vi "(A) Test-Sequence-Control (SubVI).vi"(0 "TEST MODE":bool, 1 "START":bool, 2 "STOP":bool, 3 "Hold-Step?":bool, 4 "Command Next Step":bool, 5 "Step Control":T2={"Step Description"="Description", "Step Time Target"=10.0, "Step Time Unit"=0, "Step End Action"=0} {"Step End Action" items=["Go to Next Step", "Loop to 1st Step", "Loop to Step N", "Stop Test Mode", "Stop Program"]; "Step Time Target" min=0.0 format="%#.1f"; "Step Time Unit" items=["sec", "min", "hr"]}, 7 "Step # Limit":i32=50, 9 "Loop # Limit":i32=10, 11 "Step N":i32=3, 13 "Initialize":bool) -> (14 "Output Values":T1={"Manual-Mode-Active?"=FALSE, "Test-Mode-Active?"=FALSE, "STEP-COMPLETE"=FALSE, "Test Description"="Manual Mode - Press Start to Begin\r\r", "Step-Time"="", "Step Text"="", "Loop Text"="", "Step Number"=-1, "Loop Number"=0}, 15 "Display":string="Manual Mode - Press Start to Begin", 16 "Step Number":i32=-1, 17 "Loop Number":i32, 18 "TEST MODE ACTIVE?":bool, 19 "STOP-PROGRAM":bool)   [LabVIEW 2010]
panel:
  # "Blake Otting - Ecolab\nCreated 5/28/07\nUpdated 2/4/11 (Rev 10.3)"
  # "Step Time Target"
  # "Units"
  # "Step End Action"
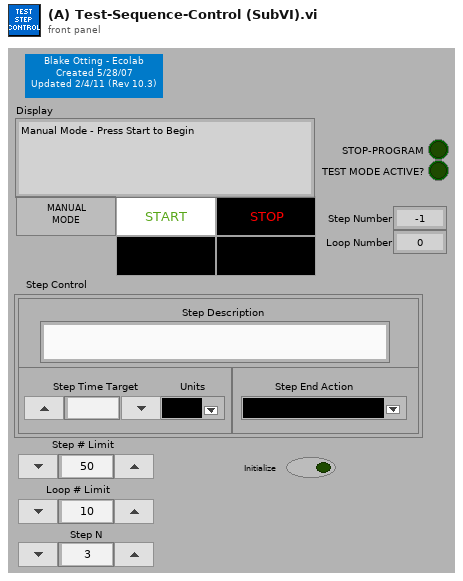
[diagram p1: front panel]
types:
  T1 = cluster{"Manual-Mode-Active?":bool, "Test-Mode-Active?":bool, "STEP-COMPLETE":bool, "Test Description":string, "Step-Time":string, "Step Text":string, "Loop Text":string, "Step Number":i32, "Loop Number":i32}
  T2 = cluster{"Step Description":string, "Step Time Target":dbl, "Step Time Unit":u16, "Step End Action":u16}
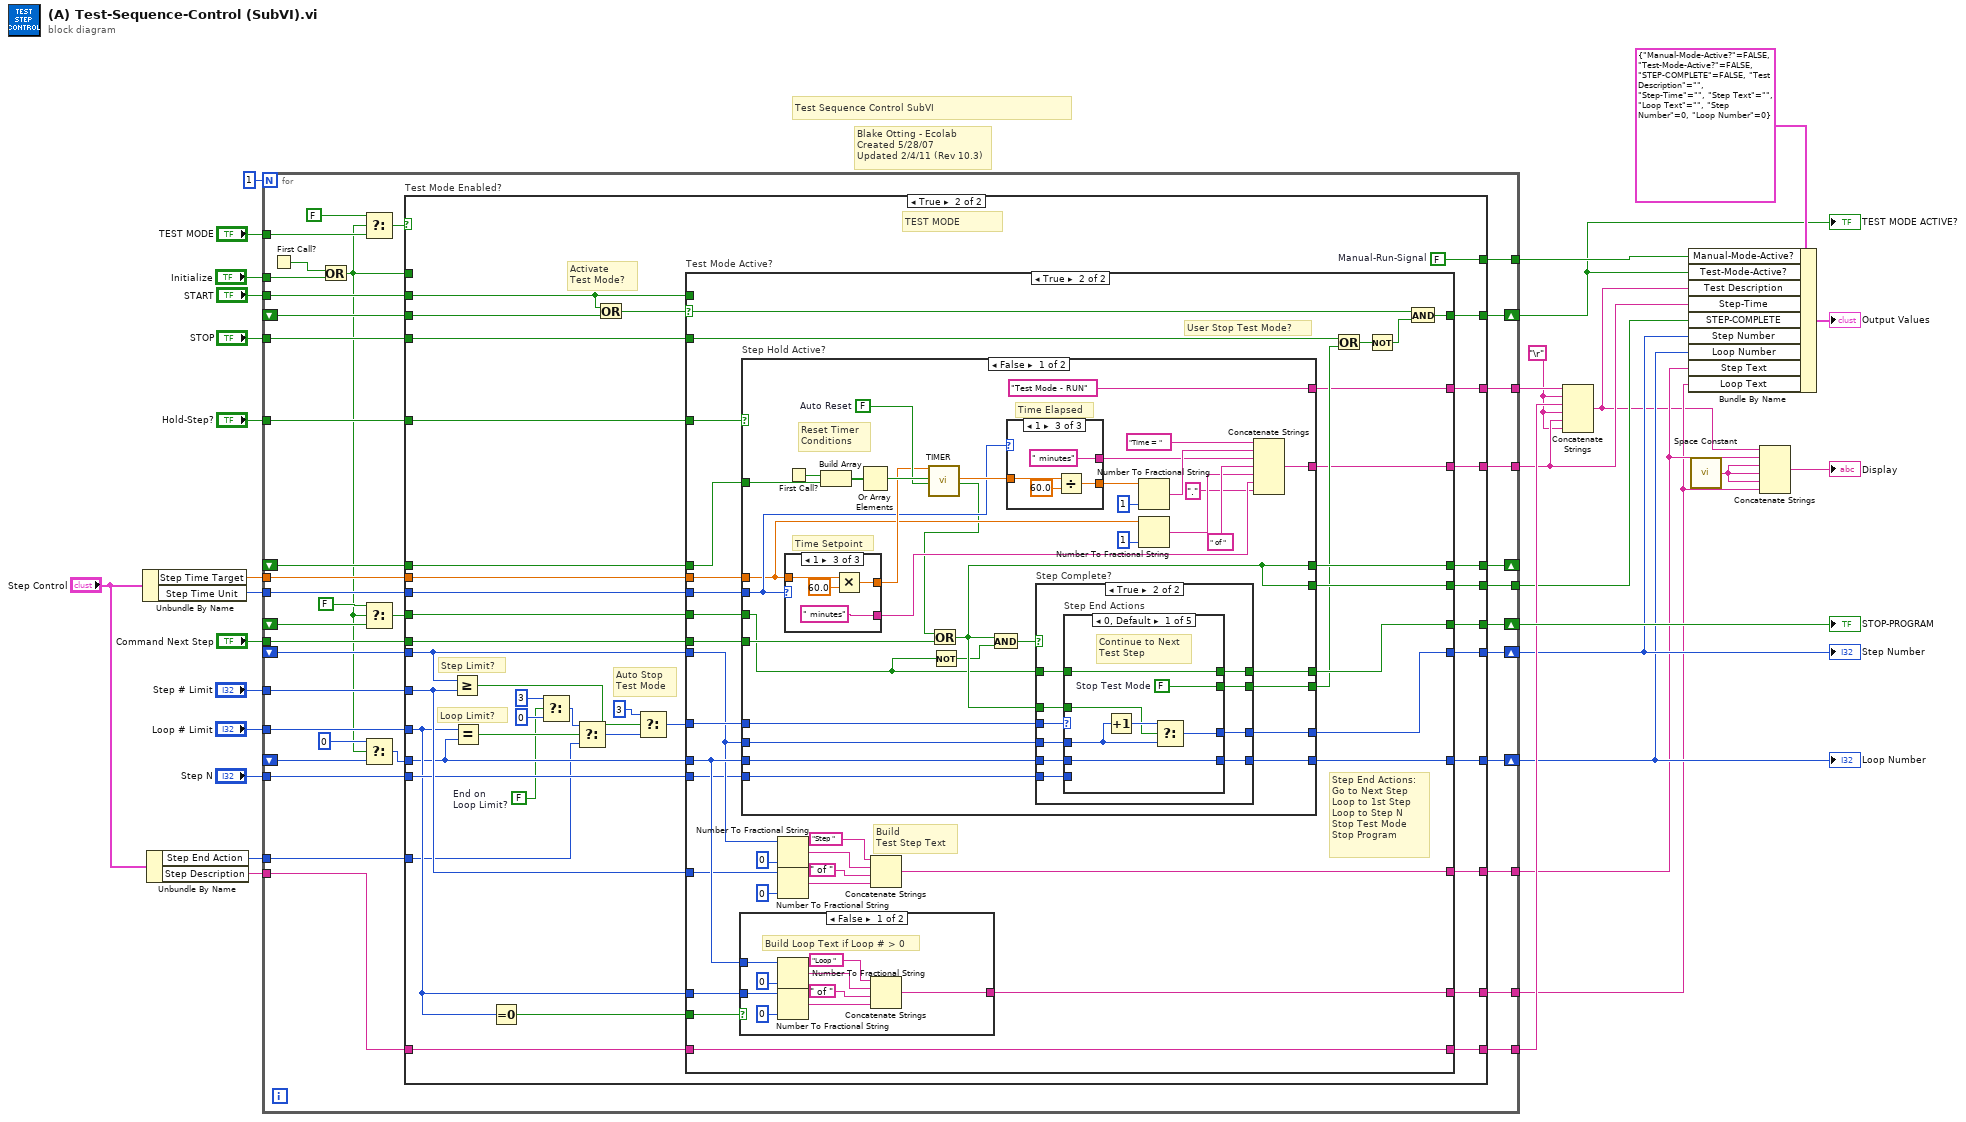
[diagram p0: block diagram]
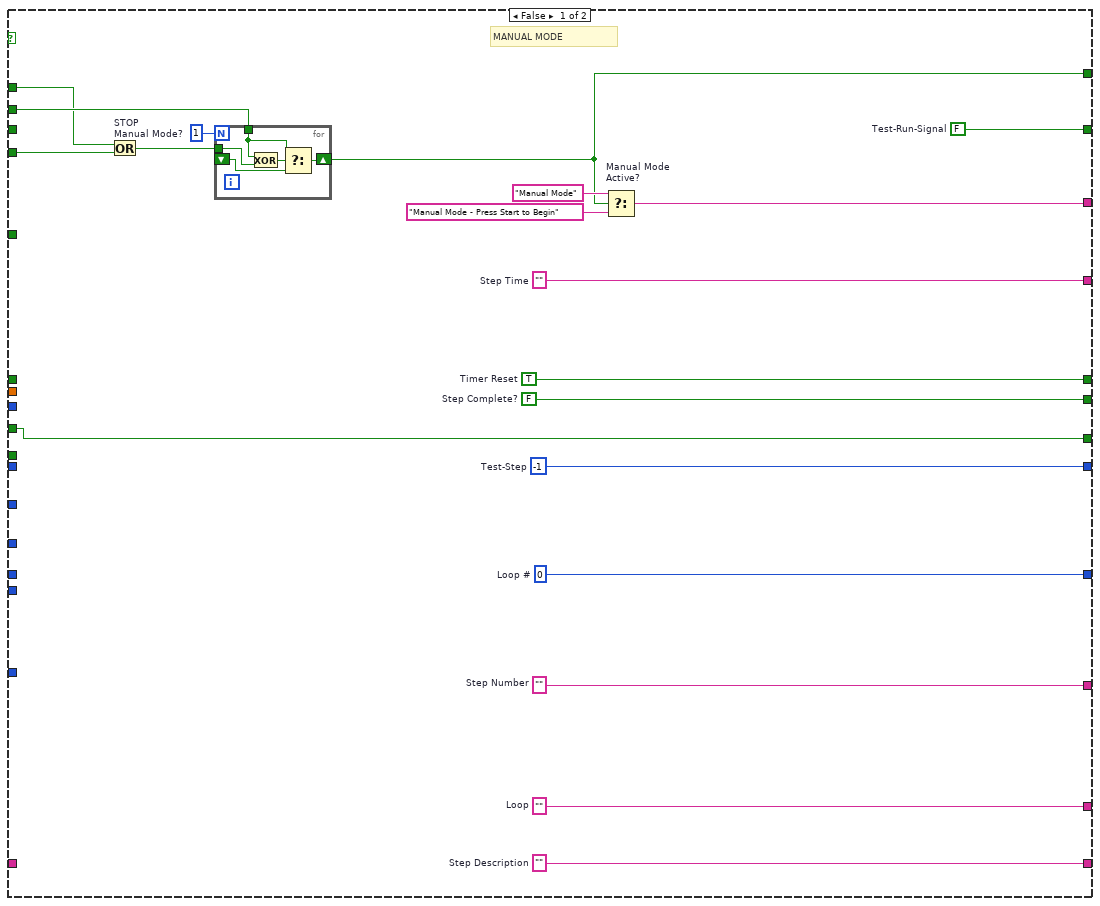
[diagram p2: hidden frame]
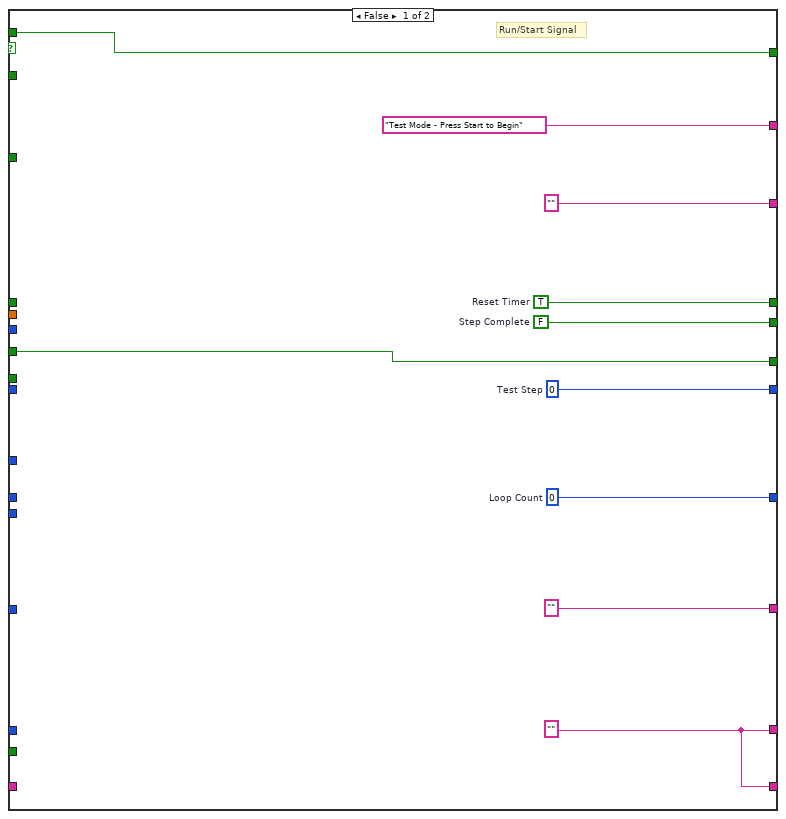
[diagram p3: hidden frame]
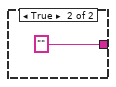
[diagram p4: hidden frame]
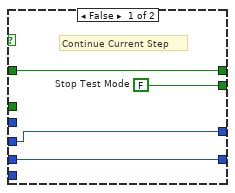
[diagram p5: hidden frame]
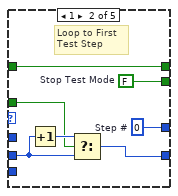
[diagram p6: hidden frame]
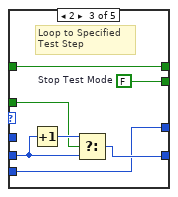
[diagram p7: hidden frame]
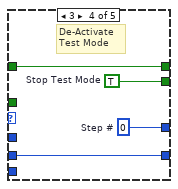
[diagram p8: hidden frame]
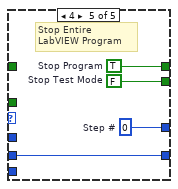
[diagram p9: hidden frame]
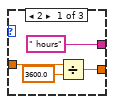
[diagram p10: hidden frame]
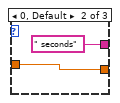
[diagram p11: hidden frame]
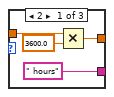
[diagram p12: hidden frame]
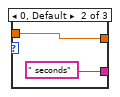
[diagram p13: hidden frame]
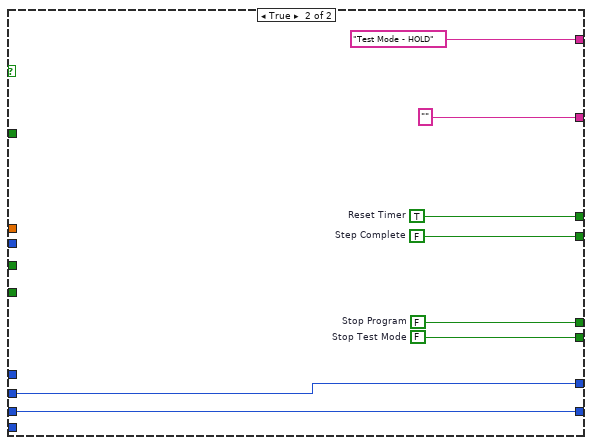
[diagram p14: hidden frame]
diagram:
  w4 = "\r"
  # "Test Sequence Control SubVI"
  # "Blake Otting - Ecolab\nCreated 5/28/07\nUpdated 2/4/11 (Rev 10.3)"
  n1 = Unbundle By Name("Step Control") -> ("Step Time Target"=w24:dbl, "Step Time Unit"=w25:u16)
  n2 = Unbundle By Name("Step Control") -> ("Step End Action"=w27:u16, "Step Description"=w26:string)
  n3 = for {
    N: 1 -> [_]
    tunnel: "Command Next Step" -> [w70]
    tunnel: [w69] -> w17
    tunnel: "TEST MODE" -> [w44]
    tunnel: "START" -> [w68]
    tunnel: "STOP" -> [w67]
    tunnel: [w65] -> w12
    tunnel: "Hold-Step?" -> [w64]
    tunnel: "Step # Limit" -> [w63]
    tunnel: "Loop # Limit" -> [w62]
    tunnel: [w61] -> w9
    tunnel: [w60] -> w3
    tunnel: [w59] -> w13
    tunnel: [w53] -> w23
    tunnel: w24 -> [w52]
    tunnel: w25 -> [w51]
    tunnel: w27 -> [w50]
    tunnel: w26 -> [w49]
    shift-right: [w55] -> w11
    shift-left: _ -> [w48]
    shift-right: [w54] -> w10
    shift-left: _ -> [w42]
    shift-right: [w56] -> _
    shift-left: _ -> [w47]
    shift-right: [w58] -> w14
    shift-left: _ -> [w46]
    tunnel: [w57] -> w15
    tunnel: "Step N" -> [w39]
    tunnel: "Initialize" -> [w35]
    shift-right: [w66] -> w21
    shift-left: _ -> [w37]
    n4 = First Call?() -> (First Call?: T/F=w34:bool)
    n5 = Or(x=w34, y=w35) -> (x .or. y?=w33:bool)
    n6 = Select(t=FALSE, s=w33, f=w44) -> (s? t:f=w43:bool)
    n7 = Select(t=FALSE, s=w33, f=w37) -> (s? t:f=w36:bool)
    n8 = Select(t=0, s=w33, f=w42) -> (s? t:f=w40:i32)
    n9 = case "Test Mode Enabled?" shown="True" w43 {
      tunnel: w68 -> [w78 w129]
      tunnel: w67 -> [w77 w132]
      tunnel: [w72 w133] -> w53
      tunnel: w46 -> [_ w131]
      tunnel: [w89 w130] -> w58
      tunnel: [w71 w127] -> w66
      tunnel: [w88 w126] -> w65
      tunnel: w64 -> [_ w125]
      tunnel: [w87 w124] -> w55
      tunnel: [w84 w123] -> w56
      tunnel: [w86 w122] -> w54
      tunnel: w63 -> [_ w119]
      tunnel: w62 -> [_ w105]
      tunnel: [w83 w118] -> w61
      tunnel: [w82 w117] -> w60
      tunnel: [w85 w116] -> w59
      tunnel: [w73 w115] -> w57
      tunnel: w47 -> [_ w114]
      tunnel: w48 -> [_ w113]
      tunnel: w40 -> [_ w104]
      tunnel: w52 -> [_ w112]
      tunnel: w51 -> [_ w111]
      tunnel: w50 -> [_ w102]
      tunnel: w49 -> [_ w110]
      tunnel: [w81 w109] -> w69
      tunnel: w70 -> [_ w108]
      tunnel: w33 -> [w76 _]
      tunnel: w39 -> [_ w107]
      tunnel: w36 -> [w71 w100]
      frame False {
        w81 = ""  # Step Description
        w82 = ""  # Loop
        w83 = ""  # Step Number
        w84 = TRUE  # Timer Reset
        w85 = ""  # Step Time
        w86 = 0  # Loop #
        w87 = -1  # Test-Step
        w88 = FALSE  # Step Complete?
        w89 = FALSE  # Test-Run-Signal
        # "MANUAL MODE"
        n10 = Or "STOP\nManual Mode?"(x=w76, y=w77) -> (x .or. y?=w80:bool)
        n11 = for {
          N: 1 -> [_]
          tunnel: w78 -> [w93]
          shift-right: [w91] -> w73
          shift-left: _ -> [w92]
          tunnel: w80 -> [w90]
          n12 = Exclusive Or(1:w90, 2:w93) -> (0:w94:bool)
          n13 = Select(t=w93, s=w94, f=w92) -> (s? t:f=w91:bool)
        }
        n14 = Select "Manual Mode\nActive?"(t="Manual Mode", s=w73, f="Manual Mode - Press Start to Begin") -> (s? t:f=w72:string)
      }
      frame True {
        w95 = FALSE  # End on Loop Limit?
        w115 = FALSE  # Manual-Run-Signal
        # "Loop Limit?"
        # "TEST MODE"
        # "Activate\nTest Mode?"
        # "Auto Stop\nTest Mode"
        # "Step Limit?"
        n15 = Greater Or Equal?(x=w113, y=w119) -> (x >= y?=w106:bool)
        n16 = Equal?(x=w105, y=w104) -> (x = y?=w103:bool)
        n17 = Equal To 0?(x=w105) -> (x = 0?=w120:bool)
        n18 = Select(t=u16 3, s=w95, f=u16 0) -> (s? t:f=w96:u16)
        n19 = Select(t=w96, s=w103, f=w102) -> (s? t:f=w101:u16)
        n20 = Or(x=w129, y=w131) -> (x .or. y?=w128:bool)
        n21 = Select(t=u16 3 ("element"), s=w106, f=w101) -> (s? t:f=w121:u16)
        n22 = case "Test Mode Active?" shown="True" w128 {
          selector: w128 -> [_ w178]
          tunnel: w132 -> [_ w167]
          tunnel: ["Test Mode - Press Start to Begin" w164] -> w133
          tunnel: [w142 w176] -> w130
          tunnel: w129 -> [w142 _]
          tunnel: w113 -> [_ w155]
          tunnel: [w134 w169] -> w127
          tunnel: [w141 w168] -> w126
          tunnel: w125 -> [_ w175]
          tunnel: [w140 w174] -> w124
          tunnel: [w136 w173] -> w123
          tunnel: [w139 w172] -> w122
          tunnel: w104 -> [_ w162]
          tunnel: w114 -> [_ w171]
          tunnel: w121 -> [_ w170]
          tunnel: w120 -> [_ w163]
          tunnel: w105 -> [_ w161]
          tunnel: w119 -> [_ w154]
          tunnel: ["" w153] -> w118
          tunnel: [w135 w151] -> w117
          tunnel: w112 -> [_ w150]
          tunnel: w111 -> [_ w149]
          tunnel: ["" w148] -> w116
          tunnel: w110 -> [_ w147]
          tunnel: [w135 w147] -> w109
          tunnel: w108 -> [_ w146]
          tunnel: w107 -> [_ w145]
          tunnel: w100 -> [w134 w144]
          frame False {
            w136 = TRUE  # Reset Timer
            w135 = ""
            w139 = 0  # Loop Count
            w140 = 0  # Test Step
            w141 = FALSE  # Step Complete
            # "Run/Start Signal"
          }
          frame True {
            # "Step End Actions:\nGo to Next Step\nLoop to 1st Step\nLoop to Step N\nStop Test Mode\nStop Program"
            # "Build \nTest Step Text"
            # "User Stop Test Mode?"
            n23 = case shown="False" w163 {
              tunnel: w162 -> [w185 _]
              tunnel: w161 -> [w183 _]
              tunnel: [w179 ""] -> w151
              frame False {
                # "Build Loop Text if Loop # > 0"
                n24 = Number To Fractional String(number=w185, precision (6)=i16 0 ("width (-)")) -> (F-format string=w184:string)  [unwired: 2 out]
                n25 = Number To Fractional String(number=w183, precision (6)=i16 0 ("width (-)")) -> (F-format string=w182:string)  [unwired: 2 out]
                n26 = Concatenate Strings("Loop ", w184, " of ", w182) -> (w179:string)
              }
              frame True {
              }
            }
            n27 = case "Step Hold Active?" shown="False" w175 {
              tunnel: [w223 w289] -> w174
              tunnel: [w193 w294] -> w173
              tunnel: [w193 w293] -> w168
              tunnel: w155 -> [w218 w289]
              tunnel: [w217 w292] -> w172
              tunnel: w162 -> [w216 w292]
              tunnel: w171 -> [w215 _]
              tunnel: w170 -> [w214 _]
              tunnel: [w213 w288] -> w169
              tunnel: [w212 w291] -> w166
              tunnel: ["Test Mode - RUN" "Test Mode - HOLD"] -> w164
              tunnel: w150 -> [w196 _]
              tunnel: w149 -> [w198 _]
              tunnel: [w197 ""] -> w148
              tunnel: w146 -> [w195 _]
              tunnel: w145 -> [w194 _]
              tunnel: w144 -> [w191 _]
              frame False {
                w221 = FALSE  # Auto Reset
                # "Time Elapsed"
                # "Time Setpoint"
                # "Reset Timer\nConditions"
                n28 = First Call?() -> (First Call?: T/F=w220:bool)
                n29 = case "Time Target & Units" shown="1" w198 {
                  tunnel: [" hours" " seconds" " minutes"] -> w200
                  tunnel: [w278 w281 w284] -> w206
                  tunnel: w196 -> [w279 w281 w285]
                  frame 2 {
                    n30 = Multiply(x=w279, y=3600.0) -> (x*y=w278:dbl)
                  }
                  frame 0, Default {
                  }
                  frame 1 {
                    n31 = Multiply(x=w285, y=60.0) -> (x*y=w284:dbl)
                  }
                }
                n32 = Build Array(w220, w215) -> (w219:bool[])
                n33 = Or Array Elements(Boolean array=w219) -> (logical OR=w222:bool)
                n34 = call "TIMER"("Time Target (s)"=w206, "Reset"=w222, "Auto Reset"=w221) -> ("Elapsed Time (s)"=w210:dbl, "Time has Elapsed"=w189:bool)  [unwired: 2 in, 13 out]
                n35 = Or(x=w189, y=w195) -> (x .or. y?=w193:bool)
                n36 = Not(x=w191) -> (.not. x?=w190:bool)
                n37 = And(x=w193, y=w190) -> (x .and. y?=w192:bool)
                n38 = case "Time Target & Units" shown="1" w198 {
                  tunnel: w210 -> [w270 w272 w276]
                  tunnel: [w268 w272 w274] -> w205
                  tunnel: [" hours" " seconds" " minutes"] -> w203
                  frame 2 {
                    n39 = Divide(x=w270, y=3600.0) -> (x/y=w268:dbl)
                  }
                  frame 0, Default {
                  }
                  frame 1 {
                    n40 = Divide(x=w276, y=60.0) -> (x/y=w274:dbl)
                  }
                }
                n41 = case "Step Complete?" shown="True" w192 {
                  tunnel: [w226 w237] -> w223
                  tunnel: w218 -> [w226 w236]
                  tunnel: [w225 w235] -> w217
                  tunnel: w216 -> [w225 w234]
                  tunnel: w214 -> [_ w233]
                  tunnel: [w224 w232] -> w213
                  tunnel: [w227 w231] -> w212
                  tunnel: w193 -> [_ w230]
                  tunnel: w194 -> [_ w229]
                  tunnel: w191 -> [w224 w228]
                  frame False {
                    w227 = FALSE  # Stop Test Mode
                    # "Continue Current Step"
                  }
                  frame True {
                    n42 = case "Step End Actions" shown="0, Default" w233 {
                      tunnel: [w241 w251 w253 w262 w265] -> w237
                      tunnel: [w238 w245 w252 w259 w266] -> w232
                      tunnel: [w240 w250 w256 w260 w263] -> w235
                      tunnel: w236 -> [w243 _ _ _ _]
                      tunnel: w230 -> [w242 w248 w255 _ _]
                      tunnel: w234 -> [w240 w247 w254 w260 w263]
                      tunnel: [w239 w246 w258 w261 w264] -> w231
                      tunnel: w229 -> [_ _ w253 _ _]
                      tunnel: w228 -> [w238 w245 w252 w259 _]
                      frame 0, Default {
                        w239 = FALSE  # Stop Test Mode
                        # "Continue to Next\nTest Step"
                        n43 = Increment(x=w243) -> (x+1=w244:i32)
                        n44 = Select(t=w244, s=w242, f=w243) -> (s? t:f=w241:i32)
                      }
                      frame 1 {
                        w246 = FALSE  # Stop Test Mode
                        w251 = 0  # Step #
                        # "Loop to First\nTest Step"
                        n45 = Increment(x=w247) -> (x+1=w249:i32)
                        n46 = Select(t=w249, s=w248, f=w247) -> (s? t:f=w250:i32)
                      }
                      frame 2 {
                        w258 = FALSE  # Stop Test Mode
                        # "Loop to Specified\nTest Step"
                        n47 = Increment(x=w254) -> (x+1=w257:i32)
                        n48 = Select(t=w257, s=w255, f=w254) -> (s? t:f=w256:i32)
                      }
                      frame 3 {
                        w261 = TRUE  # Stop Test Mode
                        w262 = 0  # Step #
                        # "De-Activate \nTest Mode"
                      }
                      frame 4 {
                        w264 = FALSE  # Stop Test Mode
                        w265 = 0  # Step #
                        w266 = TRUE  # Stop Program
                        # "Stop Entire\nLabVIEW Program"
                      }
                    }
                  }
                }
                n49 = Number To Fractional String(number=w205, precision (6)=i16 1 ("width (-)")) -> (F-format string=w204:string)  [unwired: 2 out]
                n50 = Number To Fractional String(number=w196, precision (6)=i16 1 ("width (-)")) -> (F-format string=w201:string)  [unwired: 2 out]
                n51 = Concatenate Strings("Time = ", w204, w203, " of ", w201, w200, "." ("string")) -> (w197:string)
              }
              frame True {
                w288 = FALSE  # Stop Program
                w291 = FALSE  # Stop Test Mode
                w293 = FALSE  # Step Complete
                w294 = TRUE  # Reset Timer
              }
            }
            n52 = Number To Fractional String(number=w155, precision (6)=i16 0 ("width (-)")) -> (F-format string=w159:string)  [unwired: 2 out]
            n53 = Number To Fractional String(number=w154, precision (6)=i16 0 ("width (-)")) -> (F-format string=w158:string)  [unwired: 2 out]
            n54 = Concatenate Strings("Step ", w159, " of ", w158) -> (w153:string)
            n55 = Or(x=w167, y=w166) -> (x .or. y?=w165:bool)
            n56 = Not(x=w165) -> (.not. x?=w177:bool)
            n57 = And(x=w178, y=w177) -> (x .and. y?=w176:bool)
          }
        }
      }
    }
  }
  "STOP-PROGRAM" <- w21
  "Step Number" <- w11
  "Loop Number" <- w10
  "TEST MODE ACTIVE?" <- w14
  n58 = Concatenate Strings(w23, w4, w17, w4, w13, w4) -> (w1:string)
  n59 = Bundle By Name(cluster=T1 {"Manual-Mode-Active?"=FALSE, "Test-Mode-Active?"=FALSE, "STEP-COMPLETE"=FALSE, "Test Description"="", "Step-Time"="", "Step Text"="", "Loop Text"="", "Step Number"=0, "Loop Number"=0}, "Manual-Mode-Active?"=w15, "Test-Mode-Active?"=w14, "Test Description"=w1, "Step-Time"=w13, "STEP-COMPLETE"=w12, "Step Number"=w11, "Loop Number"=w10, "Step Text"=w9, "Loop Text"=w3) -> (→"Output Values":T1)
  n60 = call <vilib>:"Space Constant.vi"() -> ("String"=w2:string)
  n61 = Concatenate Strings(w1, w9, w2, w2, w2, w3) -> (→"Display":string)
